vi "fpga_1DAC_sine_and_1ADC_W_risingedge_R_trailingedge.vi"() -> ()   [LabVIEW 2018]
uses:
  <vilib>/rvi/FXPMathLib/FxpSinAndCos/subVIs/nifxpmath_SinAndCos_SimConfig.ctl
  <vilib>/rvi/Emulation/niFpgaGetClockAttributes.vi
  <vilib>/rvi/Emulation/niFpgaSctlEmulationGetInTimedLoop.vi
  <vilib>/rvi/Emulation/niFpgaEmulationReportErrorSimple.vi
  <vilib>/rvi/eio/common/nirviEmuTemplateMethod_errors.vi
  <vilib>/rvi/FXPMathLib/FxpSinAndCos/simVIs/DllFxpSinAndCosTemp_sub.vi
  <vilib>/rvi/Emulation/niFpgaCriticalErrorInLSC.vi
  <vilib>/eio/EIONode/EIONode.xnode
  <vilib>/rvi/FXPMathLib/FxpSinAndCos/XNode/nifxpmath_SinAndCos.xnode
panel:
  out "DAC 1 write":bool[](array[boolean])=[FALSE, TRUE, TRUE, TRUE, TRUE, TRUE, TRUE, TRUE, TRUE, TRUE, TRUE, TRUE, TRUE, TRUE, TRUE, TRUE]
  out "ADC CH1 read":bool[](array[boolean])=[FALSE, FALSE, FALSE, TRUE, TRUE, TRUE, FALSE, TRUE, FALSE, TRUE, FALSE, FALSE, FALSE, TRUE, FALSE, FALSE]
  in  "datapoints/cycle":u16=100
  in  "amplitude (V)":fxp<+/-,9,5>=1.0
  in  "offset (V)":fxp<+/-,9,5>
  in  "ADC CH1 write":bool[](array[boolean])=[FALSE, FALSE, FALSE, FALSE, FALSE, TRUE, FALSE, FALSE, FALSE, FALSE, FALSE, FALSE, FALSE, FALSE, FALSE, FALSE]
  in  "delay (us)":u32=40000
  in  "Stop":bool
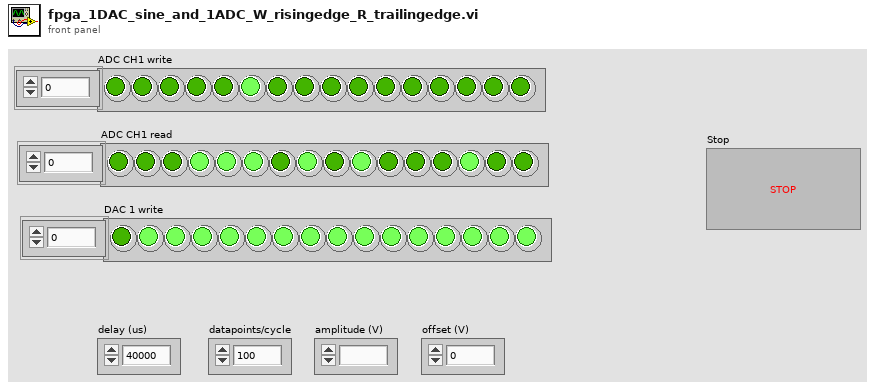
[diagram p1: front panel]
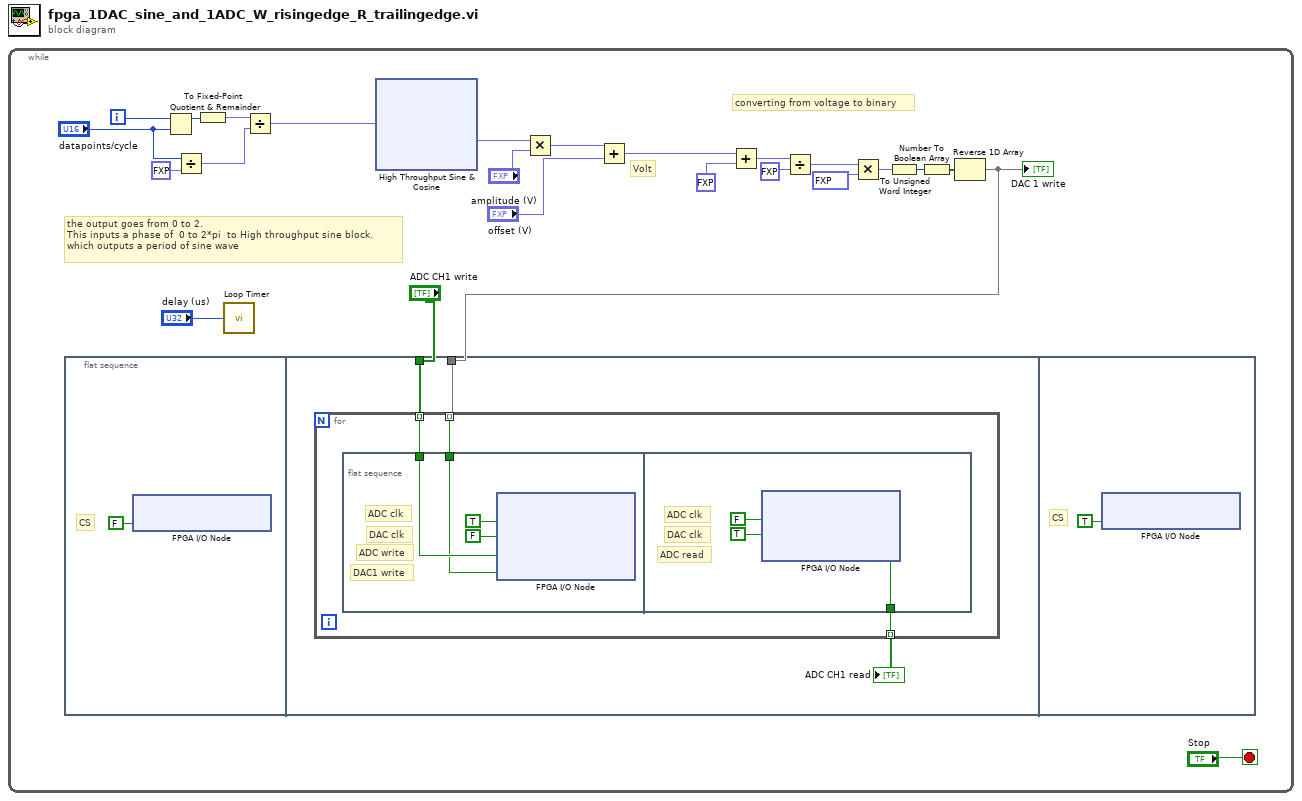
[diagram p0: block diagram]
diagram:
  n1 = while {
    i -> [w14]
    stop <- "Stop" stop-if-true
    # "converting from voltage to binary"
    # "Volt"
    # "the output goes from 0 to 2.\nThis inputs a phase of  0 to 2*pi  to High throughput sine block.\nwhich outputs a period of sine wave"
    n2 = flat-sequence {
      tunnel: w1 -> [w58]
      tunnel: "ADC CH1 write" -> [w57]
      frame #0 {
        # "CS"
        n3 = xnode "FPGA I/O Node"("ConnectorA/DIO4"=FALSE) -> ()  [unwired: 1 in, 1 out]
      }
      frame #1 {
        n4 = for {
          tunnel: w58 -> [w61] mode=indexing
          tunnel: w57 -> [w60] mode=indexing
          tunnel: [w59] -> w56 mode=indexing
          n5 = flat-sequence {
            tunnel: w61 -> [w62]
            tunnel: w60 -> [w63]
            tunnel: [w66] -> w59
            frame #0 {
              # "DAC1 write"
              # "ADC write"
              # "DAC clk"
              # "ADC clk"
              n6 = xnode "FPGA I/O Node"("ConnectorA/DIO3"=TRUE, "ConnectorA/DIO5"=FALSE, "ConnectorA/DIO2"=w63, "ConnectorA/DIO6"=w62) -> ()  [unwired: 4 in, 4 out]
            }
            frame #1 {
              # "ADC read"
              # "DAC clk"
              # "ADC clk"
              n7 = xnode "FPGA I/O Node"("ConnectorA/DIO3"=FALSE, "ConnectorA/DIO5"=TRUE) -> ("ConnectorA/DIO1"=w66:bool)  [unwired: 3 in, 3 out]
            }
          }
        }
        "ADC CH1 read" <- w56
      }
      frame #2 {
        # "CS"
        n8 = xnode "FPGA I/O Node"("ConnectorA/DIO4"=TRUE) -> ()  [unwired: 1 in, 1 out]
      }
    }
    n9 = Quotient & Remainder(x=w14, y="datapoints/cycle") -> (x-y*floor(x/y)=w13:i32)  [unwired: 1 out]
    n10 = Divide(x="datapoints/cycle", y=fxp<+,1,2> 2.0) -> (x/y=w5:fxp<+,17,15>)
    n11 = To Fixed-Point(number=w13) -> (fixed-point=w7:fxp<+/-,16,12>)  [unwired: 1 in]
    n12 = call "Loop Timer"("Count(Ticks)"="delay (us)") -> ()  [unwired: 1 out]
    n13 = Divide(x=w7, y=w5) -> (x/y=w12:fxp<+/-,33,14>)
    n14 = xnode "High Throughput Sine & Cosine"("x (pi)"=w12) -> ("sin(x)"=w11:fxp<+/-,16,2>)  [unwired: 1 out]
    n15 = Multiply(x=w11, y="amplitude (V)") -> (x*y=w16:fxp<+/-,25,7>)
    n16 = Add(x=w16, y="offset (V)") -> (x+y=w10:fxp<+/-,25,7>)
    n17 = Add(x=w10, y=fxp<+,3,4> 10.0) -> (x+y=w22:fxp<+/-,25,7>)
    n18 = Divide(x=w22, y=fxp<+,3,5> 20.0) -> (x/y=w9:fxp<+/-,26,3>)
    n19 = Multiply(x=w9, y=fxp<+,16,16> 65535.0) -> (x*y=w8:fxp<+/-,42,19>)
    n20 = To Unsigned Word Integer(number=w8) -> (unsigned 16bit integer=w20:u16)
    n21 = Number To Boolean Array(number=w20) -> (Boolean array=w19:bool[])
    n22 = Reverse 1D Array(array=w19) -> (reversed array=w1:bool[])
    "DAC 1 write" <- w1
  }
